vi "1.1_Test.vi"   [LabVIEW 2017]
uses:
  <vilib>/addons/_JKI Toolkits/Caraya/classes/Assert/Assert Equal Value_Variant.vi
  <vilib>/addons/_JKI Toolkits/Caraya/classes/Test/Test.lvclass
  <vilib>/addons/_JKI Toolkits/Caraya/classes/Assert/Assert.lvclass
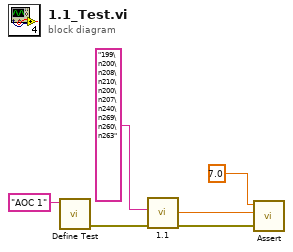
[diagram p0: block diagram]
diagram:
  n1 = call <vilib>:"Define Test.vi"("Label (VI Title)"="AOC 1") -> ("error out"=w5:errorcluster)  [unwired: 10 in]
  n2 = call "1.1.vi"("error in (no error)"=w5, "input"="199\n200\n208\n210\n200\n207\n240\n269\n260\n263") -> ("error out"=w4:errorcluster, "Out"=w2:dbl)  [unwired: 8 in]
  n3 = call-poly <vilib>:"Assert.vi"("error in (no error)"=w4, "Y"=w2, "X"=7.0) -> ()  [unwired: 8 in, 1 out]
